vi "Main_6_Dynamic_9234[FPGA].vi"() -> ()   [LabVIEW 2017]
uses:
  <vilib>/LabVIEW Targets/FPGA/cRIO/shared/nicrio_ModuleControls/nicrio_cRIO-9232_ConfigModeRing.ctl
  <vilib>/rvi/Emulation/niFpgaGetClockAttributes.vi
  <vilib>/rvi/Emulation/niFpgaSctlEmulationGetInTimedLoop.vi
  <vilib>/rvi/Emulation/niFpgaEmulationReportErrorSimple.vi
  <vilib>/rvi/Emulation/niFpgaProcessEmulError.vi
  <vilib>/rvi/eio/common/nirviEmuTemplateMethod_errors.vi
  <vilib>/rvi/interface/RandomDataEmulation/niFpgaRandomDataHandleErrors.vi
  <vilib>/rvi/Emulation/niFpgaCriticalErrorInLSC.vi
  <vilib>/eio/EIONode/EIONode.xnode
  <vilib>/rvi/DataTransferAndStorage/Container/XNode/niFpgaContainer.xnode
  <vilib>/rvi/interface/RandomDataEmulation/nirviRandomDataFpgaReadWriteTemplate.vi
  <vilib>/addons/InsightCM/Devices/Shared/Cms/Fpga/Acquisition/source/subVIs/VibAPI/BOP_VibAPI_6.lvlib
panel:
  out "Chassis Temperature":sgl
  in  "Custom Scale Intercept":sgl[](array[numeric])=[0.0, 0.0, 0.0, 0.0, 0.0, 0.0, 0.0, 0.0, 0.0, 0.0, 0.0, 0.0, 0.0, 0.0, 0.0, 0.0, 0.0, 0.0, 0.0, 0.0, 0.0, 0.0, 0.0, 0.0, 0.0, 0.0, 0.0, 0.0, 0.0, 0.0, 0.0, 0.0]
  out "FPGA Error":errorcluster
  out "Finished":bool
  in  "Stop":bool
  out "Module Underflow":bool
  out "DMA FIFO Full":bool
  out "Chan Count":bool
  out "Acq Loop Ticks":u32
  out "Short Circuit Chan Array":bool[](array[boolean])
  out "Open Loop Chan Array":bool[](array[boolean])
  out "First Read":bool
  in  "Total Avail Channels":i32=4
  in  "Data Rate [S/s]":u32=1280
  in  "Custom Scale Slope":sgl[](array[numeric])=[0.0, 0.0, 0.0, 0.0, 0.0, 0.0, 0.0, 0.0, 0.0, 0.0, 0.0, 0.0, 0.0, 0.0, 0.0, 0.0, 0.0, 0.0, 0.0, 0.0, 0.0, 0.0, 0.0, 0.0, 0.0, 0.0, 0.0, 0.0, 0.0, 0.0, 0.0, 0.0]
  in  "Acquisition Type":enum16{"Finite Samples", "Continuous Samples"}(ring)
  in  "Samps per Chan [Finite]":i32=5120
  in  "Input Config Array":T1[](array[typedef])=[0, 0, 0, 0, 0, 0, 0, 0, 0, 0, 0, 0, 0, 0, 0, 0, 0, 0, 0, 0, 0, 1, 1, 1, 0, 0, 0, 0, 0, 0, 0, 0] items=["AC Coupled", "DC Coupled", "IEPE AC Coupled"]
  in  "Number of Modules":i16=1
  in  "Enable Chan Array":bool[](array[boolean])=[FALSE, FALSE, FALSE, FALSE, FALSE, FALSE, FALSE, FALSE, FALSE, FALSE, FALSE, FALSE, FALSE, FALSE, FALSE, FALSE, FALSE, FALSE, FALSE, FALSE, FALSE, FALSE, FALSE, FALSE, FALSE, FALSE, FALSE, FALSE, FALSE, FALSE, FALSE, FALSE]
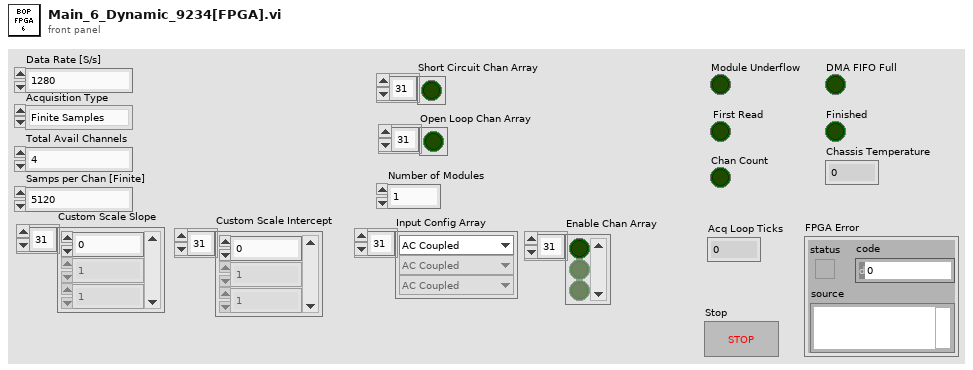
[diagram p1: front panel]
types:
  T1 = typedef "nicrio_cRIO-9232_ConfigModeRing.ctl" = u8
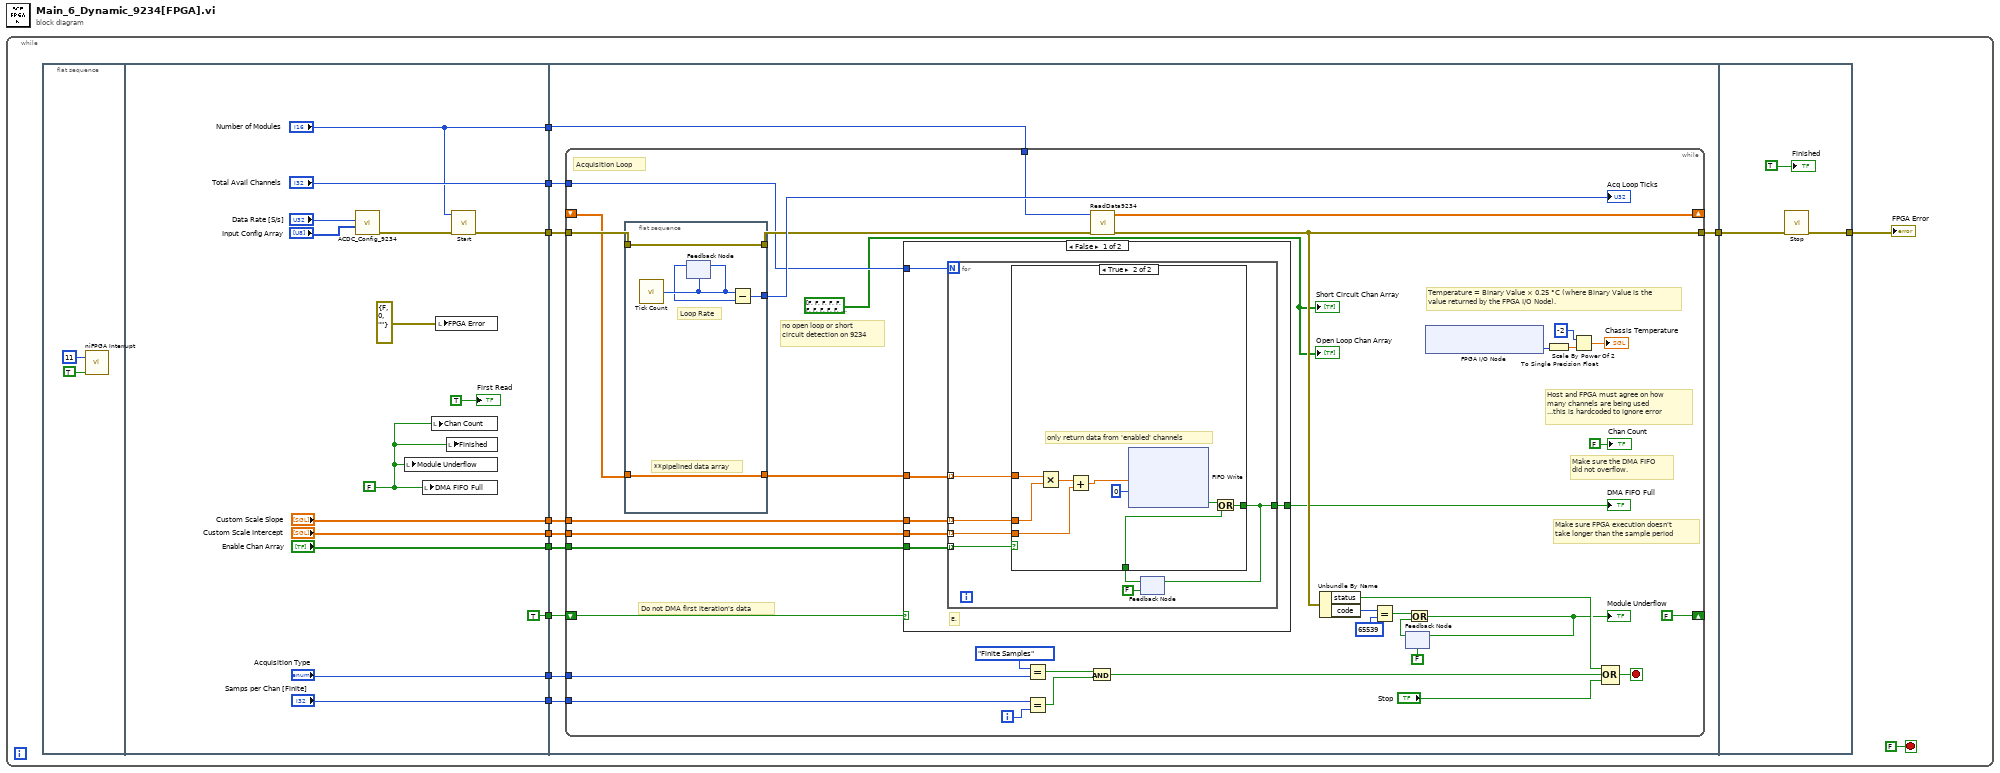
[diagram p0: block diagram]
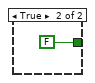
[diagram p3: hidden frame]
diagram:
  n1 = while {
    stop <- FALSE stop-if-true
    n2 = flat-sequence {
      tunnel: [w22] -> w11
      tunnel: ["Custom Scale Slope"] -> w10
      tunnel: ["Acquisition Type"] -> w9
      tunnel: ["Samps per Chan [Finite]"] -> w8
      tunnel: ["Total Avail Channels"] -> w7
      tunnel: [TRUE ("t")] -> w6
      tunnel: ["Number of Modules"] -> w4
      tunnel: ["Enable Chan Array"] -> w3
      tunnel: ["Custom Scale Intercept"] -> w1
      tunnel: w11 -> [w38]
      tunnel: w10 -> [w37]
      tunnel: w9 -> [w35]
      tunnel: w8 -> [w34]
      tunnel: w7 -> [w39]
      tunnel: w6 -> [w36]
      tunnel: [w33] -> w5
      tunnel: w4 -> [w32]
      tunnel: w3 -> [w31]
      tunnel: w1 -> [w30]
      tunnel: w5 -> [w107]
      tunnel: [w106] -> w2
      frame #0 {
        n3 = call <vilib>:"niFPGA Interrupt.vi"("Wait Until Cleared (F)"=TRUE ("Wait Until Cleared"), "IRQ Number (0)"=u8 11 ("IRQ Number")) -> ()  [unwired: 1 in]
      }
      frame #1 {
        w23 = FALSE ("Module Underflow")
        n4 = call <vilib>:"ACDC_Config_9234.vi"("Input Config Array"="Input Config Array", "Data Rate [S/s]"="Data Rate [S/s]") -> ("error out"=w20:errorcluster)  [unwired: 9 in]
        n5 = local write "Module Underflow"(w23) -> ()
        n6 = local write "DMA FIFO Full"(w23) -> ()
        n7 = local write "Chan Count"(w23) -> ()
        n8 = local write "FPGA Error"(errorcluster {"status"=FALSE, "code"=0, "source"=""} ("FPGA Error")) -> ()
        n9 = local write "Finished"(w23) -> ()
        n10 = call <vilib>:"Start.vi"("error in (no error)"=w20, "Module Config Selector"="Number of Modules") -> ("error out"=w22:errorcluster)  [unwired: 9 in]
        "First Read" <- TRUE ("First Read")
      }
      frame #2 {
        n11 = while {
          tunnel: w38 -> [w69]
          tunnel: [w70] -> w33
          tunnel: w35 -> [w72]
          tunnel: w34 -> [w71]
          shift-right: [w64] -> _
          shift-left: _ -> [w67]
          tunnel: w39 -> [w48]
          tunnel: w37 -> [w47]
          shift-right: [FALSE ("t")] -> _
          shift-left: w36 -> [w51]
          tunnel: w32 -> [w54]
          tunnel: w31 -> [w46]
          tunnel: w30 -> [w45]
          i -> [w65]
          stop <- w75 stop-if-true
          w40 = bool[] [FALSE, FALSE, FALSE, FALSE, FALSE, FALSE, FALSE, FALSE, FALSE, FALSE, FALSE, FALSE, FALSE, FALSE, FALSE, FALSE, FALSE, FALSE, FALSE, FALSE, FALSE, FALSE, FALSE, FALSE, FALSE, FALSE, FALSE, FALSE, FALSE, FALSE, FALSE, FALSE] ("Open Loop Chan Array")
          # "no open loop or short circuit detection on 9234"
          # "Temperature = Binary Value × 0.25 °C (where Binary Value is the value returned by the FPGA I/O Node)."
          # "Do not DMA first iteration's data"
          # "Acquisition Loop"
          # "Host and FPGA must agree on how \nmany channels are being used\n...this is hardcoded to ignore error"
          # "Make sure the DMA FIFO\ndid not overflow."
          # "Make sure FPGA execution doesn't\ntake longer than the sample period"
          n12 = flat-sequence {
            tunnel: [w105] -> w52
            tunnel: w69 -> [w105]
            tunnel: [w102] -> w68
            tunnel: w67 -> [w101]
            tunnel: [w101] -> w49
            frame #0 {
              # "**pipelined data array"
              # "Loop Rate"
              n13 = call "Tick Count"() -> ("Tick Count(Ticks)"=w104:u32)
              n14 = feedback-in #1(w104) -> ()
              n15 = feedback #1(w104) -> (w103:u32)
              n16 = Subtract(x=w104, y=w103) -> (x-y=w102:u32)
            }
          }
          n17 = case shown="False" w51 {
            tunnel: [w82 FALSE] -> w50
            tunnel: w47 -> [w81 _]
            tunnel: w49 -> [w80 _]
            tunnel: w48 -> [w79 _]
            tunnel: w46 -> [w78 _]
            tunnel: w45 -> [w77 _]
            frame False {
              # "E."
              n18 = for {
                N: w79 -> [_]
                tunnel: [w88] -> w82
                tunnel: w80 -> [w87] mode=indexing
                tunnel: w81 -> [w86] mode=indexing
                tunnel: w78 -> [w84] mode=indexing
                tunnel: w77 -> [w83] mode=indexing
                n19 = feedback #2(FALSE) -> (w89:bool)
                n20 = case shown="True" w84 {
                  tunnel: w89 -> [w90 w99]
                  tunnel: [w90 w98] -> w88
                  tunnel: w87 -> [_ w97]
                  tunnel: w86 -> [_ w96]
                  tunnel: w83 -> [_ w91]
                  frame False {
                  }
                  frame True {
                    # "only return data from 'enabled' channels"
                    n21 = Multiply(x=w97, y=w96) -> (x*y=w93:sgl)
                    n22 = Add(x=w93, y=w91) -> (x+y=w92:sgl)
                    n23 = xnode ("FIFO Write")("Element"=w92, "Timeout"=0) -> ("Timed Out?"=w94:bool)  [unwired: 1 in, 1 out]
                    n24 = Or(x=w94, y=w99) -> (x .or. y?=w98:bool)
                  }
                }
                n25 = feedback-in #2(w88) -> ()
              }
            }
            frame True {
            }
          }
          "DMA FIFO Full" <- w50
          n26 = Equal?(x=enum16{"Finite Samples", "Continuous Samples"}."Finite Samples" ("y"), y=w72) -> (x = y?=w58:bool)
          n27 = Equal?(x=w71, y=w65) -> (x = y?=w57:bool)
          n28 = And(x=w58, y=w57) -> (x .and. y?=w56:bool)
          n29 = call <vilib>:"ReadData9234.vi"("error in"=w52, "Module Config Selector"=w54) -> ("error out"=w70:errorcluster, "Data Array"=w64:sgl[])  [unwired: 8 in]
          n30 = Unbundle By Name(w70) -> ("status"=w63:bool, "code"=w73:i32)
          n31 = Equal?(x=w73, y=65539) -> (x = y?=w60:bool)
          n32 = feedback #3(FALSE) -> (w62:bool)
          n33 = Or(x=w60, y=w62) -> (x .or. y?=w59:bool)
          "Module Underflow" <- w59
          n34 = feedback-in #3(w59) -> ()
          n35 = xnode "FPGA I/O Node"() -> ("Chassis Temperature"=w42:i16)  [unwired: 1 in, 1 out]
          n36 = To Single Precision Float(number=w42) -> (single precision float=w44:sgl)
          n37 = Scale By Power Of 2(n=i16 -2, x=w44) -> (x*2^n=→"Chassis Temperature":sgl)
          n38 = Compound Arithmetic op=OR(w63, w56, "Stop") -> (w75:bool)
          "Chan Count" <- FALSE ("Chan Count")
          "Acq Loop Ticks" <- w68
          "Short Circuit Chan Array" <- w40
          "Open Loop Chan Array" <- w40
        }
      }
      frame #3 {
        n39 = call <vilib>:"Stop.vi"("error in (no error)"=w107) -> ("error out"=w106:errorcluster)  [unwired: 10 in]
        "Finished" <- TRUE ("Finished")
      }
    }
    "FPGA Error" <- w2
  }
